vi "Stop Test.vi"(8 "error in (no error)":errorcluster, 11 "Coverage Analyzer in":refnum<class "Coverage Analyzer.lvclass">) -> (0 "error out":errorcluster, 3 "Coverage Analyzer out":refnum<class "Coverage Analyzer.lvclass">)   [LabVIEW 2020, in "Coverage Analyzer.lvlib" / "Coverage Analyzer.lvclass"]
uses:
  Coverage Analyzer.lvclass
  Coverage Analyzer Result View/Coverage Analyzer View Data.ctl
  Coverage Analyzer.lvclass/Coverage Analyzer.ctl
  Coverage Analyzer Result View/Coverage Analyzer View.vi
  Coverage Analyzer Result View/Coverage Analyzer Result View.lvclass
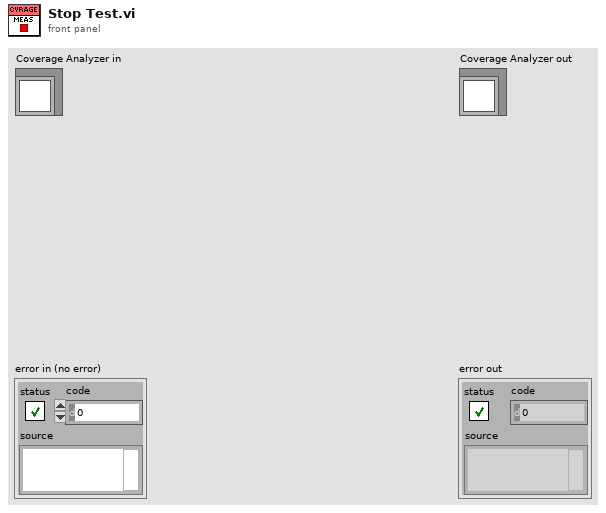
[diagram p1: front panel]
types:
  T1 = typedef "Coverage Analyzer.lvlib/Coverage Analyzer Result View.lvclass/Coverage Analyzer View Data.ctl" = cluster{"Code Coverage":map{path, dbl}}
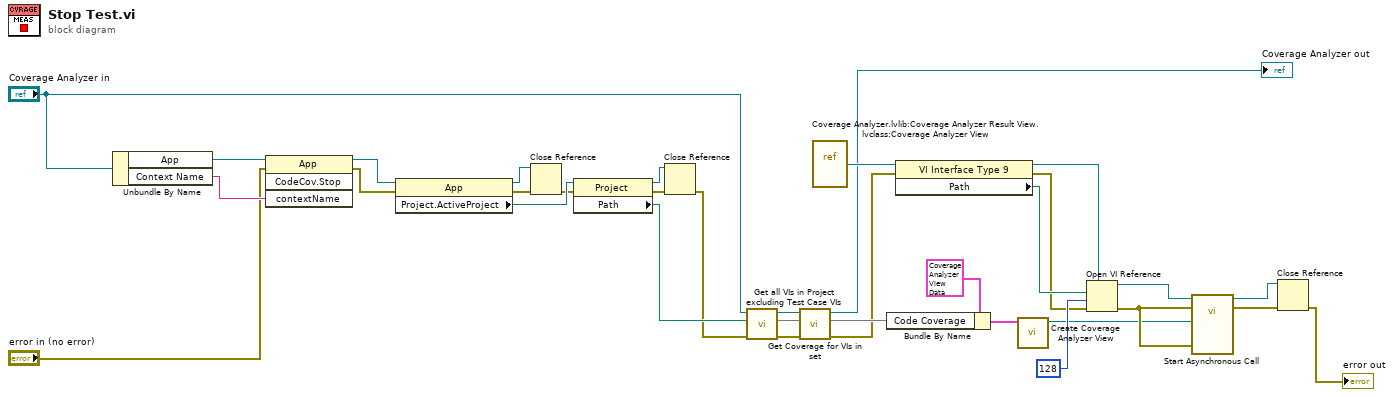
[diagram p0: block diagram]
diagram:
  n1 = Unbundle By Name("Coverage Analyzer in") -> ("App"=w33:refnum<vi>, "Context Name"=w32:string)
  n2 = invoke class="App" method="CodeCov.Stop"(reference=w33, error in="error in (no error)", "contextName"=w32) -> (reference out=w24:refnum<vi>, error out=w3:errorcluster)  [unwired: 1 in, 2 out]
  n3 = property class="App"(reference=w24, error in=w3) -> (reference out=w29:refnum<vi>, error out=w26:errorcluster, "Project.ActiveProject"=w30:refnum<vi>)
  n4 = Close Reference(reference=w29, error in (no error)=w26) -> (error out=w25:errorcluster)
  n5 = property class="Project"(reference=w30, error in=w25) -> (reference out=w28:refnum<vi>, error out=w27:errorcluster, "Path"=w6:path)
  n6 = Close Reference(reference=w28, error in (no error)=w27) -> (error out=w2:errorcluster)
  n7 = call "Get all VIs in Project excluding Test Case VIs.vi"("error in (no error)"=w2, "Path"=w6, "Coverage Analyzer in"="Coverage Analyzer in") -> ("error out"=w11:errorcluster, "VIs"=w7:set{path}, "Coverage Analyzer out"=w13:refnum<class "Coverage Analyzer.lvclass">)  [unwired: 6 in]
  n8 = call "Get Coverage for VIs in set.vi"("error in (no error)"=w11, "VIs"=w7, "Coverage Analyzer in"=w13) -> ("error out"=w10:errorcluster, "Code Coverage"=w12:map{path, dbl}, "Coverage Analyzer out"=→"Coverage Analyzer out":refnum<class "Coverage Analyzer.lvclass">)  [unwired: 6 in]
  n9 = vi-ref "Coverage Analyzer.lvlib:Coverage Analyzer Result View.lvclass:Coverage Analyzer View.vi"() -> (w16:refnum<vi>)
  n10 = Bundle By Name(cluster=T1 {"Code Coverage"={}} ("Data"), "Code Coverage"=w12) -> (w9:T1)
  n11 = property class="VI Interface Type 9"(reference=w16, error in=w10) -> (reference out=w20:refnum<vi>, error out=w18:errorcluster, "Path"=w19:path)
  n12 = call "Create Coverage Analyzer View.vi"("Coverage Analyzer Result View in"=w9) -> ("Coverage Analyzer Result View out"=w8:refnum<class "Coverage Analyzer Result View.lvclass">)  [unwired: 9 in, 1 out]
  n13 = Open VI Reference(type specifier VI Refnum (for type only)=w20, vi path=w19, options=128, error in (no error)=w18) -> (vi reference=w15:refnum<vi>, error out=w17:errorcluster)  [unwired: 2 in]
  n14 = call-by-ref "Start Asynchronous Call"(reference=w15, error in=w17, 8:"error in (no error)"=w17, "Coverage Analyzer Result View.lvclass"=w8) -> (reference out=w23:refnum<vi>, error out=w22:errorcluster)  [unwired: 9 in, 1 out]
  n15 = Close Reference(reference=w23, error in (no error)=w22) -> (error out=→"error out":errorcluster)
